vi "复制Excel表模板.vi"(11 "当前零件型号":string) -> (1 "file or folder exists?":bool caption="文件或文件夹存在？", 3 "添加的路径":path)   [LabVIEW 2014]
uses:
  Global.vi
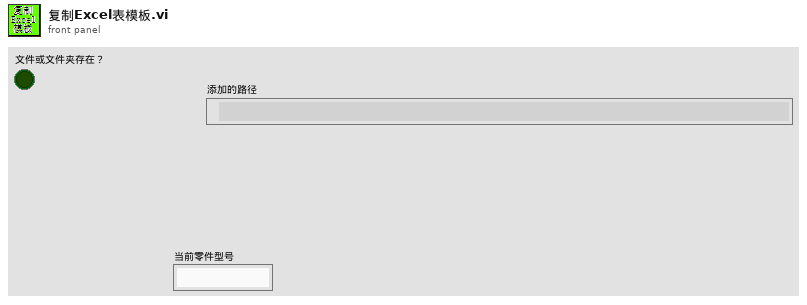
[diagram p1: front panel]
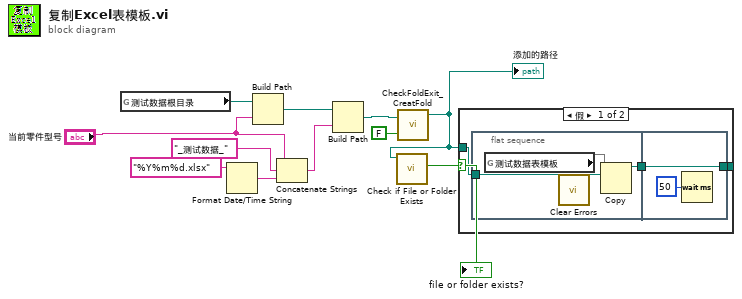
[diagram p0: block diagram]
diagram:
  n1 = global read "Global.vi" "测试数据根目录"() -> (w4:path)
  n2 = Format Date/Time String(time format string (%c)="%Y%m%d.xlsx" ("时间格式字符串(%c)")) -> (date/time string=w7:string)  [unwired: 2 in]
  n3 = Build Path(base path=w4, name or relative path="当前零件型号") -> (appended path=w5:path)
  n4 = Concatenate Strings("当前零件型号", "_测试数据_" ("名称或相对路径"), w7) -> (w8:string)
  n5 = Build Path(base path=w5, name or relative path=w8) -> (appended path=w9:path)
  n6 = call "CheckFoldExit_CreatFold.vi"("path in"=w9, "FoldOrFile¡H"=FALSE) -> ("File out"=w11:path)  [unwired: 2 out]
  "添加的路径" <- w11
  n7 = call <vilib>:"Check if File or Folder Exists.vi"("path"=w11) -> ("file or folder exists?"=w10:bool)  [unwired: 1 in, 9 out]
  "file or folder exists?" <- w10
  n8 = case shown="假" w10 {
    tunnel: w11 -> [w13 w20]
    tunnel: [w12 w20] -> _
    frame False {
      n9 = flat-sequence {
        tunnel: w13 -> [w17]
        tunnel: [w15] -> w14
        tunnel: [w19] -> w12
        tunnel: w14 -> [w19]
        frame #0 {
          n10 = global read "Global.vi" "测试数据表模板"() -> (w16)
          n11 = call <vilib>:"Clear Errors.vi"() -> ()  [unwired: 6 in, 2 out]
          n12 = Copy(10:w17, 11:w16) -> (3:w15:path)  [unwired: 3 in, 2 out]
        }
        frame #1 {
          n13 = Wait (ms)(milliseconds to wait=u32 50 ("等待时间（毫秒）")) -> ()  [unwired: 1 out]
        }
      }
    }
    frame True {
    }
  }
